vi "Write Page Button List Properties.vi"(8 "error in (no error)":errorcluster, 10 "Button List Properties":T1[](array[typedef]), 11 ".NET Refnum in":refnum<k24>) -> (0 "error out":errorcluster, 3 ".NET Refnum out":refnum<k24>)   [LabVIEW 2015, in "Configuration Tool.lvlib"]
uses:
  Configuration Tool.lvlib
  NationalInstruments.VeriStand.XMLReader
  Custom Device Type Defs/ButtonLists Properties.ctl
  XML Controls/Path Cluster.ctl
  XML Controls/Button Type.ctl
  XML Controls/Dependency three item small.ctl
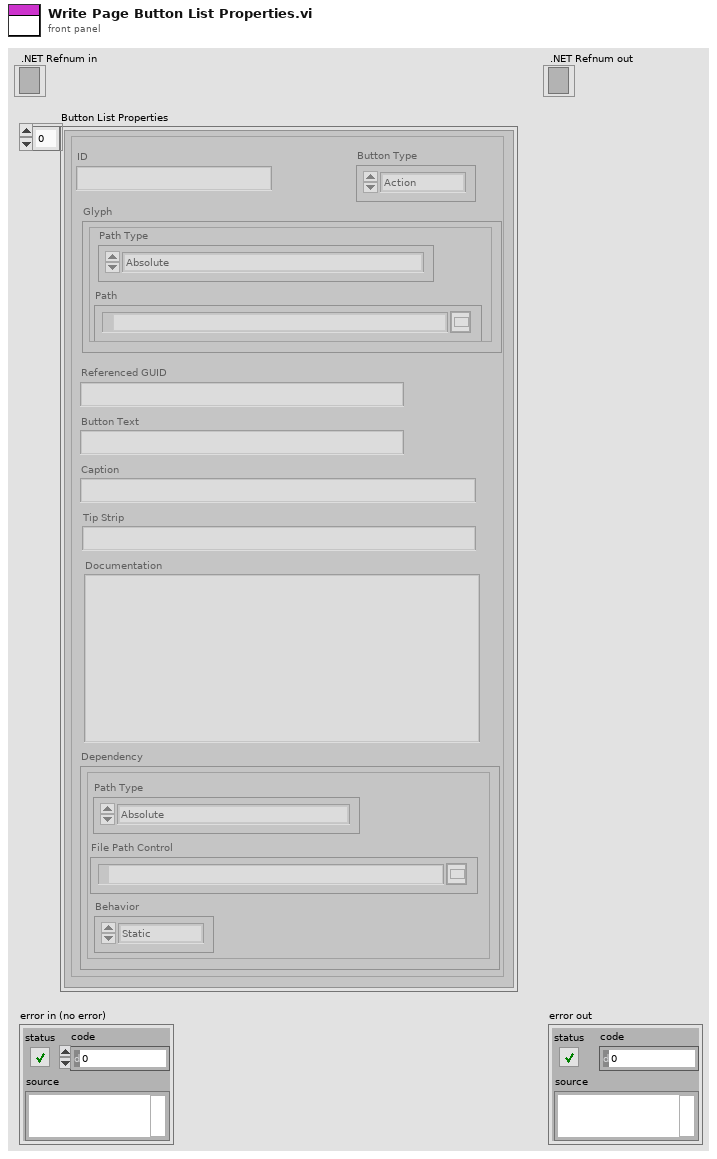
[diagram p1: front panel]
types:
  T1 = typedef "ButtonLists Properties.ctl" = cluster{"ID":string, "Glyph":T2, "Button Type":T3, "Referenced GUID":string, "Button Text":string, "Caption":string, "Tip Strip":string, "Documentation":string, "Dependency":T4}
  T2 = typedef "Configuration Tool.lvlib/Path Cluster.ctl" = cluster{"Path":path, "Path Type":enum16{"Absolute", "To Base", "To Common Doc Dir", "To Application Data Dir"}}
  T3 = typedef "Configuration Tool.lvlib/Button Type.ctl" = enum16{"Action", "Dialog", "Page", "Notification", "Separator"}
  T4 = typedef "Configuration Tool.lvlib/Dependency three item small.ctl" = cluster{"File Path Control":path, "Path Type":enum16{"Absolute", "To Base", "To Common Doc Dir", "To Application Data Dir"}, "Behavior":enum16{"Static", "Dynamic"}}
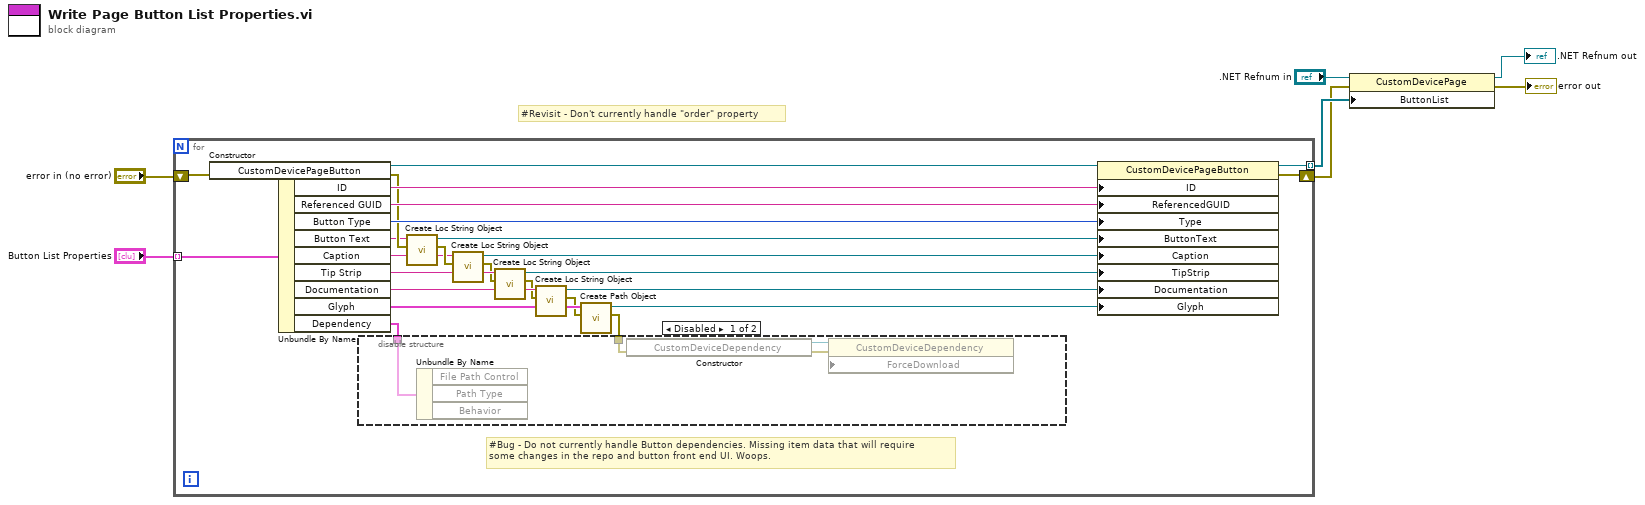
[diagram p0: block diagram]
diagram:
  # "#Revisit - Don't currently handle \"order\" property"
  n1 = for {
    tunnel: "Button List Properties" -> [w32] mode=indexing
    shift-right: [w9] -> w4
    shift-left: "error in (no error)" -> [w31]
    tunnel: [w8] -> w6 mode=indexing
    # "#Bug - Do not currently handle Button dependencies. Missing item data that will require\nsome changes in the repo and button front end UI. Woops."
    n2 = constructor class="CustomDevicePageButton"(error in=w31) -> (reference out=w30:refnum<k24>, error out=w26:errorcluster)  [unwired: 2 in, 1 out]
    n3 = Unbundle By Name(w32) -> ("ID"=w29:string, "Referenced GUID"=w28:string, "Button Type"=w27:T3, "Button Text"=w25:string, "Caption"=w22:string, "Tip Strip"=w20:string, "Documentation"=w18:string, "Glyph"=w14:T2, "Dependency"=w11:T4)
    n4 = call "Create Loc String Object.vi"("error in (no error)"=w26, "Name"=w25) -> ("error out"=w23:errorcluster, ".NET Refnum out"=w24:refnum<k24>)  [unwired: 8 in]
    n5 = call "Create Loc String Object.vi"("error in (no error)"=w23, "Name"=w22) -> ("error out"=w19:errorcluster, ".NET Refnum out"=w21:refnum<k24>)  [unwired: 8 in]
    n6 = call "Create Loc String Object.vi"("error in (no error)"=w19, "Name"=w20) -> ("error out"=w17:errorcluster, ".NET Refnum out"=w16:refnum<k24>)  [unwired: 8 in]
    n7 = call "Create Loc String Object.vi"("error in (no error)"=w17, "Name"=w18) -> ("error out"=w13:errorcluster, ".NET Refnum out"=w15:refnum<k24>)  [unwired: 8 in]
    n8 = call "Create Path Object.vi"("error in (no error)"=w13, "Path Info"=w14) -> ("error out"=w10:errorcluster, ".NET Refnum out"=w12:refnum<k24>)  [unwired: 8 in]
    n9 = disable-structure shown="Disabled" {
      disable-tunnel: w11 -> [w36 _]
      disable-tunnel: w10 -> [w35 _]
      frame Disabled {
        n10 = Unbundle By Name(w36) -> ()  [unwired: 3 out]
        n11 = constructor class="CustomDeviceDependency"(error in=w35) -> (reference out=w33:refnum<k24>, error out=w34:errorcluster)  [unwired: 2 in, 1 out]
        n12 = property class="CustomDeviceDependency" props=["ForceDownload"](reference=w33, error in=w34) -> ()  [unwired: 1 in, 2 out]
      }
      frame Enabled {
      }
    }
    n13 = property class="CustomDevicePageButton"(reference=w30, "ID"=w29, "ReferencedGUID"=w28, "Type"=w27, "ButtonText"=w24, "Caption"=w21, "TipStrip"=w16, "Documentation"=w15, "Glyph"=w12) -> (reference out=w8:refnum<k24>, error out=w9:errorcluster)  [unwired: 1 in]
  }
  n14 = property class="CustomDevicePage"(reference=".NET Refnum in", error in=w4, "ButtonList"=w6) -> (reference out=→".NET Refnum out":refnum<k24>, error out=→"error out":errorcluster)
